vi "FlatToRichrfcontrol_RFDCSendWaveformResponse.vi"(5 "OutputClusterType":T1, 11 "InputCluster":T2) -> (3 "OutputCluster":T1)   [LabVIEW 2024, in "FlexSDR_gRPC_client.lvlib"]
uses:
  FlexSDR_gRPC_client.lvlib
  rfcontrol_RFDCSendWaveformResponse_Flat.ctl
  rfcontrol_RFDCSendWaveformResponse.ctl
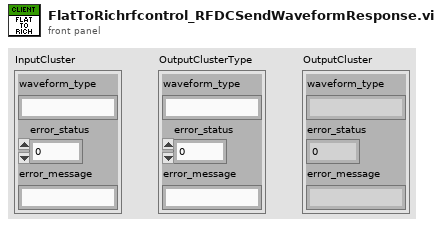
[diagram p1: front panel]
types:
  T1 = typedef "FlexSDR_gRPC_client.lvlib/rfcontrol_RFDCSendWaveformResponse.ctl" = cluster{"waveform_type":string, "error_status":i32, "error_message":string}
  T2 = typedef "FlexSDR_gRPC_client.lvlib/rfcontrol_RFDCSendWaveformResponse_Flat.ctl" = cluster{"waveform_type":string, "error_status":i32, "error_message":string}
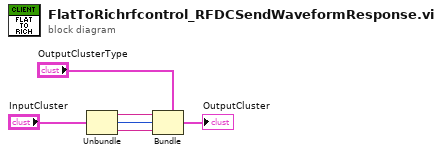
[diagram p0: block diagram]
diagram:
  n1 = Unbundle "Unbundle"("InputCluster") -> ("waveform_type"=w3:string, "error_status"=w2:i32, "error_message"=w1:string)
  n2 = Bundle "Bundle"(cluster="OutputClusterType", "waveform_type"=w3, "error_status"=w2, "error_message"=w1) -> (→"OutputCluster":T1)
